vi "SP - low click.vi"(7 "Control Label":string, 8 "error in (no error)":errorcluster, 9 "subpanel":refnum<vi>, 10 "subVI":refnum<vi>, 11 "VI with Focus":refnum<vi>) -> (0 "error out":errorcluster, 3 "return value":string)   [LabVIEW 2020, in "ui-testing.lvlib"]
uses:
  ui-testing.lvlib
  User32.dll
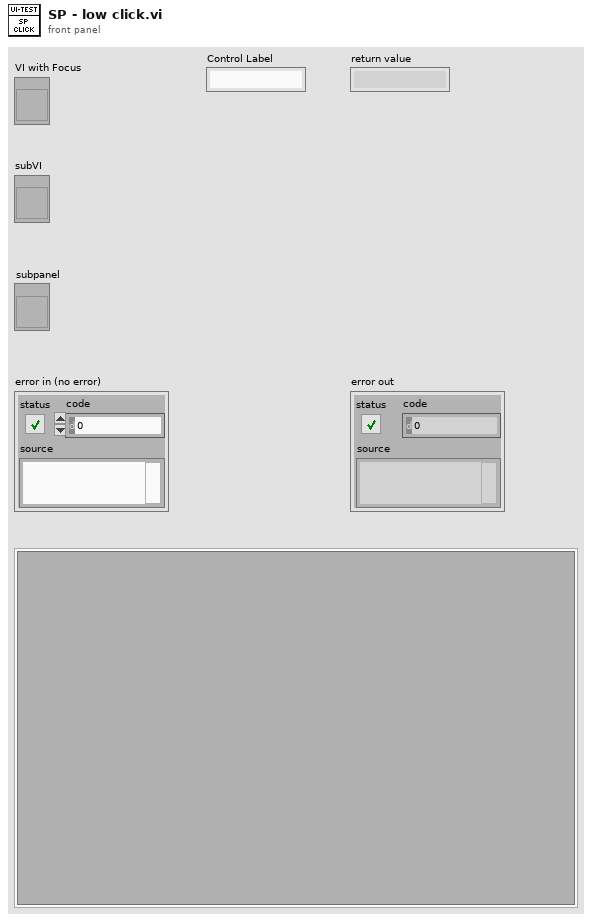
[diagram p1: front panel]
types:
  T1 = typedef "LVPositionTypeDef.ctl" = cluster{"Left":i32, "Top":i32}
  T2 = typedef "LVRectTypeDef.ctl" = cluster{"left":i16, "top":i16, "right":i16, "bottom":i16}
  T3 = typedef "LVPointTypeDef.ctl" = cluster{"Horizontal":i16, "Vertical":i16}
  T4 = typedef "LVBoundsTypeDef.ctl" = cluster{"Width":u32, "Height":u32}
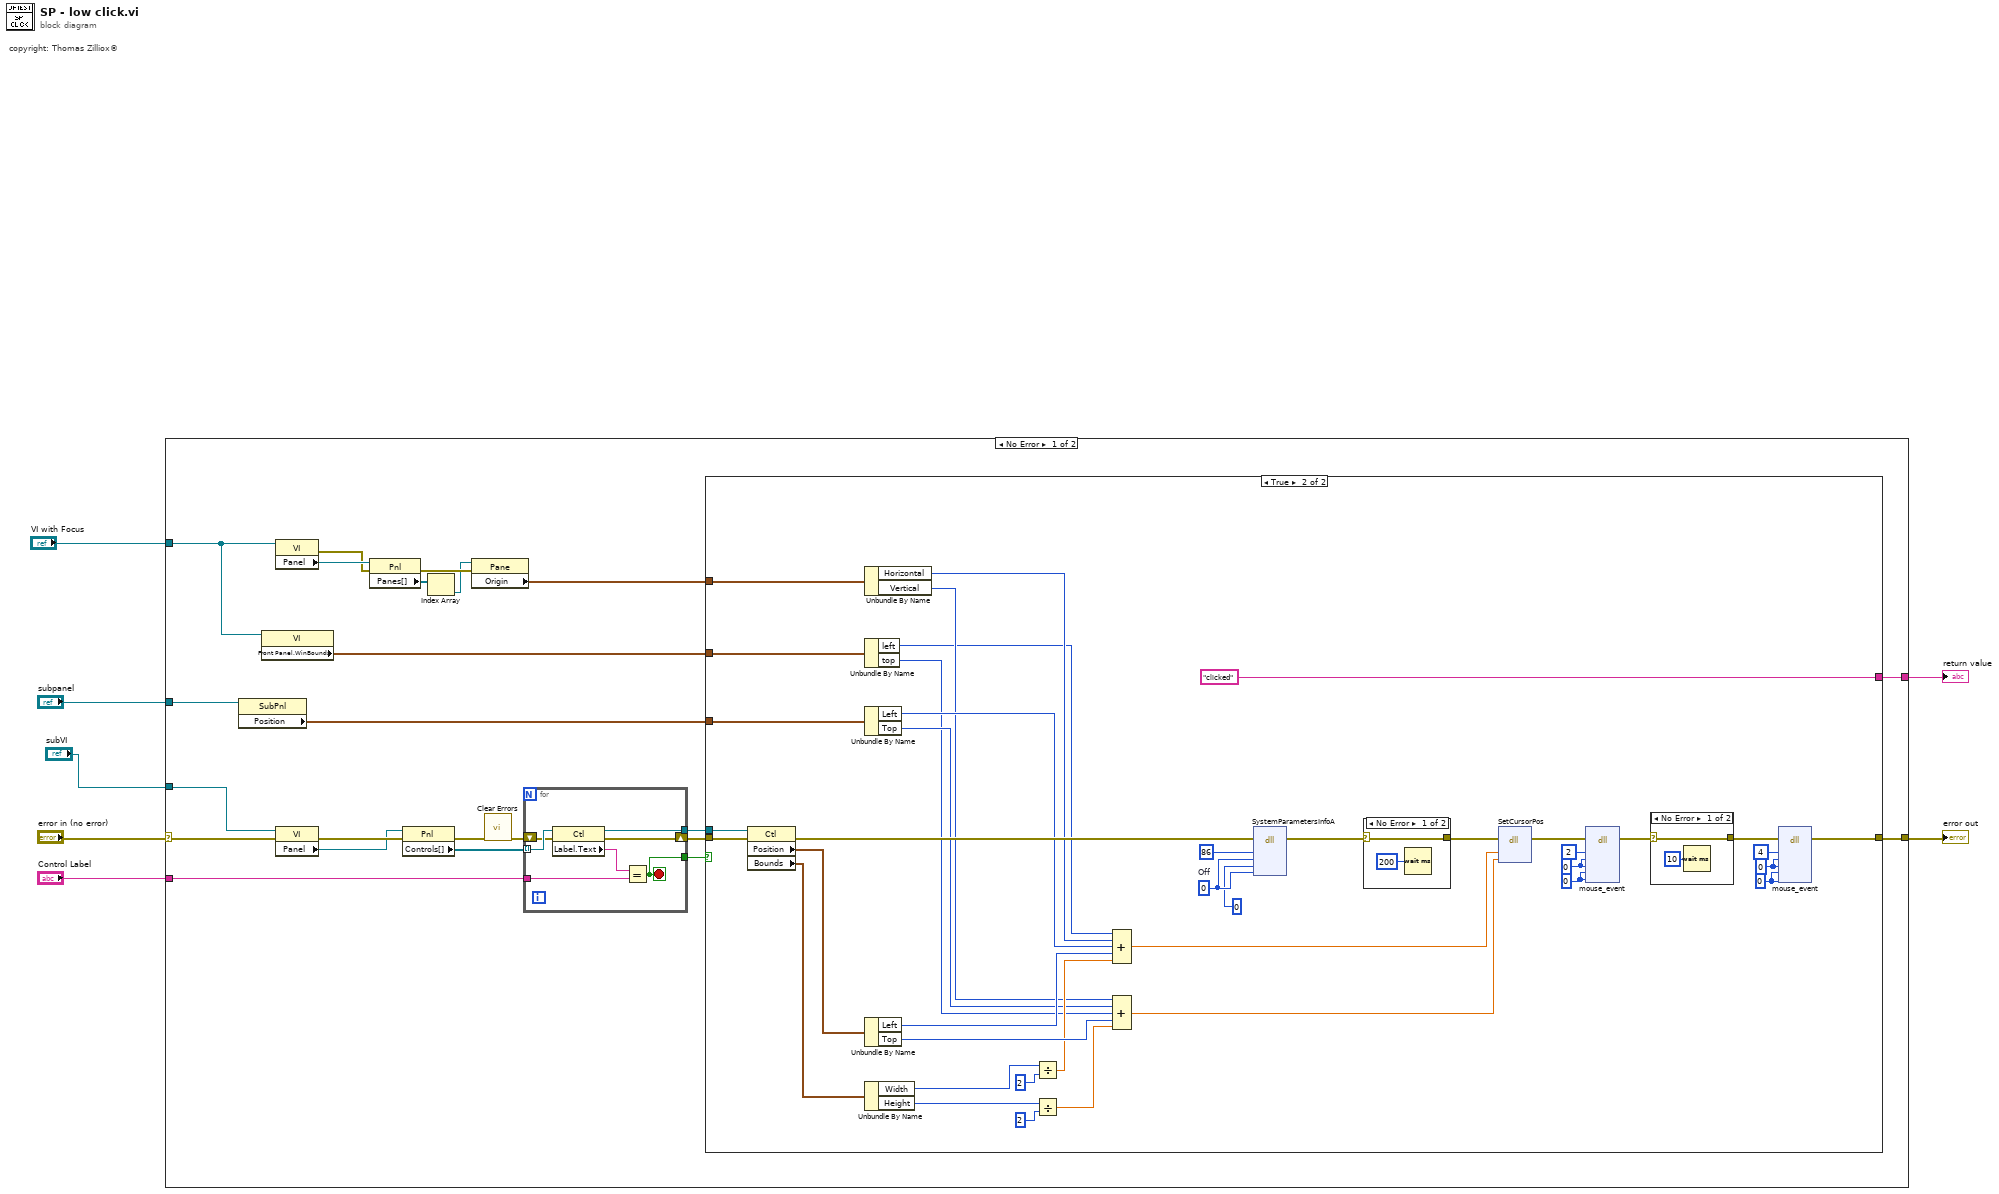
[diagram p0: block diagram]
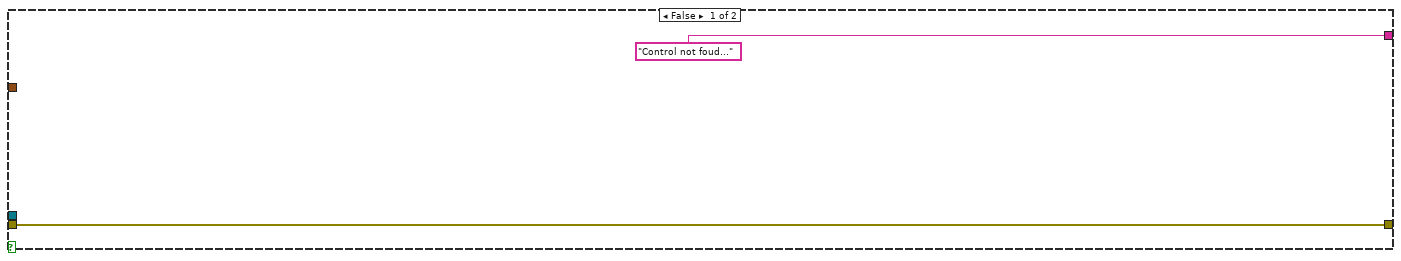
[diagram p2: hidden frame]
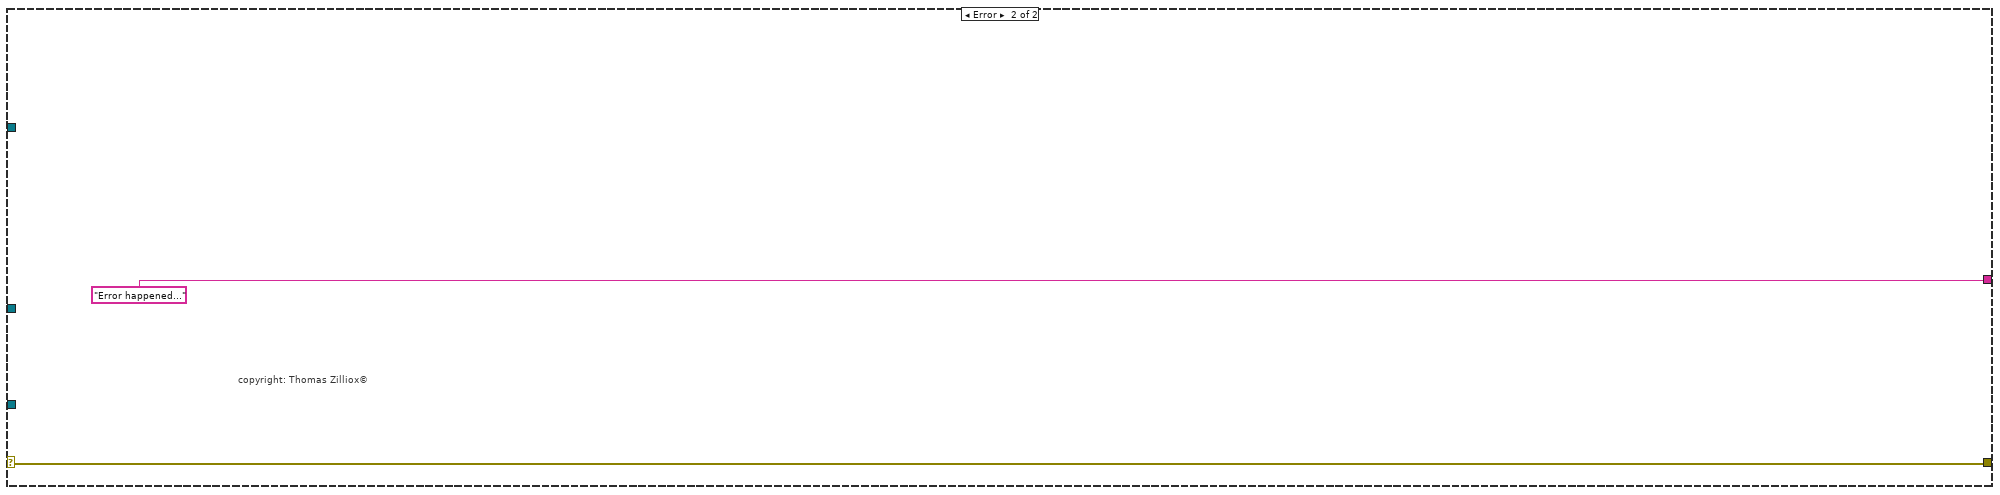
[diagram p5: hidden frame]
diagram:
  # "copyright: Thomas Zilliox©"
  n1 = case shown="No Error" "error in (no error)" {
    selector: "error in (no error)" -> [w12 w87]
    tunnel: [w13 w87] -> w6
    tunnel: "Control Label" -> [w16 _]
    tunnel: [w14 "Error happened..."] -> w4
    tunnel: "subVI" -> [w19 _]
    tunnel: "VI with Focus" -> [w18 _]
    tunnel: "subpanel" -> [w17 _]
    frame No Error {
      n2 = property class="SubPnl"(reference=w17) -> ("Position"=w11:T1)  [unwired: 1 in, 2 out]
      n3 = property class="VI"(reference=w18) -> ("Front Panel.WinBounds"=w8:T2)  [unwired: 1 in, 2 out]
      n4 = property class="VI"(reference=w18) -> (error out=w10:errorcluster, "Panel"=w20:refnum<vi>)  [unwired: 1 in, 1 out]
      n5 = property class="VI"(reference=w19, error in=w12) -> (error out=w27:errorcluster, "Panel"=w24:refnum<vi>)  [unwired: 1 out]
      n6 = property class="Pnl"(reference=w20, error in=w10) -> (error out=w23:errorcluster, "Panes[]"=w22:refnum<vi>[])  [unwired: 1 out]
      n7 = property class="Pnl"(reference=w24, error in=w27) -> (error out=w29:errorcluster, "Controls[]"=w30:refnum<vi>[])  [unwired: 1 out]
      n8 = Index Array(array=w22) -> (element=w21:refnum<vi>)  [unwired: 1 in]
      n9 = property class="Pane"(reference=w21, error in=w23) -> ("Origin"=w9:T3)  [unwired: 2 out]
      n10 = call <vilib>:"Clear Errors.vi"("error in (no error)"=w29) -> ("error out"=w28:errorcluster)  [unwired: 5 in, 1 out]
      n11 = for {
        tunnel: w30 -> [w85] mode=indexing
        tunnel: w16 -> [w83]
        tunnel: [w82] -> w26
        shift-right: [w80] -> w25
        shift-left: w28 -> [w81]
        tunnel: [w79] -> w15
        stop <- w79 stop-if-true
        n12 = property class="Ctl"(reference=w85, error in=w81) -> (reference out=w82:refnum<vi>, error out=w80:errorcluster, "Label.Text"=w84:string)
        n13 = Equal?(x=w84, y=w83) -> (x = y?=w79:bool)
      }
      n14 = case shown="True" w15 {
        tunnel: w26 -> [_ w72]
        tunnel: w25 -> [w31 w71]
        tunnel: ["Control not foud..." ("VI Name") "clicked" ("VI Name")] -> w14
        tunnel: [w31 w33] -> w13
        tunnel: w11 -> [_ w51]
        tunnel: w9 -> [_ w48]
        tunnel: w8 -> [_ w45]
        frame False {
        }
        frame True {
          w39 = 0 ("dwExtraInfo")
          w40 = u32 0 ("dwExtraInfo")
          w38 = 0 ("dwExtraInfo")
          w37 = u32 0 ("dwExtraInfo")
          w70 = u32 0  # Off
          n15 = property class="Ctl"(reference=w72, error in=w71) -> (error out=w52:errorcluster, "Position"=w63:T1, "Bounds"=w62:T4)  [unwired: 1 out]
          n16 = Unbundle By Name(w48) -> ("Horizontal"=w47:i16, "Vertical"=w46:i16)
          n17 = Unbundle By Name(w45) -> ("left"=w44:i16, "top"=w43:i16)
          n18 = Unbundle By Name(w51) -> ("Left"=w50:i32, "Top"=w49:i32)
          n19 = Unbundle By Name(w63) -> ("Left"=w61:i32, "Top"=w59:i32)
          n20 = Unbundle By Name(w62) -> ("Width"=w60:u32, "Height"=w58:u32)
          n21 = Divide(x=w60, y=u32 2) -> (x/y=w57:dbl)
          n22 = Divide(x=w58, y=u32 2) -> (x/y=w55:dbl)
          n23 = Compound Arithmetic op=ADD(w44, w47, w50, w61, w57) -> (w65:dbl)
          n24 = Compound Arithmetic op=ADD(w46, w49, w43, w59, w55) -> (w64:dbl)
          n25 = dll-call lib="User32.dll" fn="SystemParametersInfoA" label="Terminate power-off mode"(error in=w52, "uiAction"=u32 86 ("SPI_GETPOWEROFFACTIVE"), "uiParam"=w70, "pvParam"=0, "fWinIni"=w70) -> (error out=w67:errorcluster)  [unwired: 7 in, 1 out]
          n26 = case shown="No Error" w67 {
            selector: w67 -> [w76 w78]
            tunnel: [w76 w78] -> w66
            frame No Error {
              n27 = Wait (ms)(milliseconds to wait=u32 200) -> ()  [unwired: 1 out]
            }
            frame Error {
            }
          }
          n28 = dll-call lib="User32.dll" fn="SetCursorPos" label="Move mouse"(error in=w66, "dx"=w65, "dy"=w64) -> (error out=w42:errorcluster)  [unwired: 5 in, 1 out]
          n29 = dll-call lib="User32.dll" fn="mouse_event" label="Click"(error in=w42, "dwFlags"=2, "dx"=w38, "dy"=w38, "dwData"=w37, "dwExtraInfo"=w37) -> (error out=w35:errorcluster)  [unwired: 8 in, 1 out]
          n30 = case shown="No Error" w35 {
            selector: w35 -> [w73 w75]
            tunnel: [w73 w75] -> w34
            frame No Error {
              n31 = Wait (ms)(milliseconds to wait=u32 10) -> ()  [unwired: 1 out]
            }
            frame Error {
            }
          }
          n32 = dll-call lib="User32.dll" fn="mouse_event" label="Release"(error in=w34, "dwFlags"=4, "dx"=w39, "dy"=w39, "dwData"=w40, "dwExtraInfo"=w40) -> (error out=w33:errorcluster)  [unwired: 8 in, 1 out]
        }
      }
    }
    frame Error {
      # "copyright: Thomas Zilliox©"
    }
  }
  "error out" <- w6
  "return value" <- w4
